vi "Tree.vi"() -> ()   [LabVIEW 2020, in "Nominal Client.lvclass"]
uses:
  Nominal Client.lvclass
  Nominal Client.lvclass/Nominal Client.ctl
  76682c19-609f-4d4f-aff0-eacf46784d00.vi
  2ed37eeb-a64f-4a91-b3eb-4b67bea1485f.vi
  95585ae7-5aba-4d79-b365-cf4aec99f37a.vi
  384434fe-2914-4816-8bdb-9cb29dce40f3.vi
panel:
  in  "Stop wait":bool
  in  "Description":string
  in  "Timestamp Column Name":string
  in  "Dataset Name":string
  in  "File Path":path
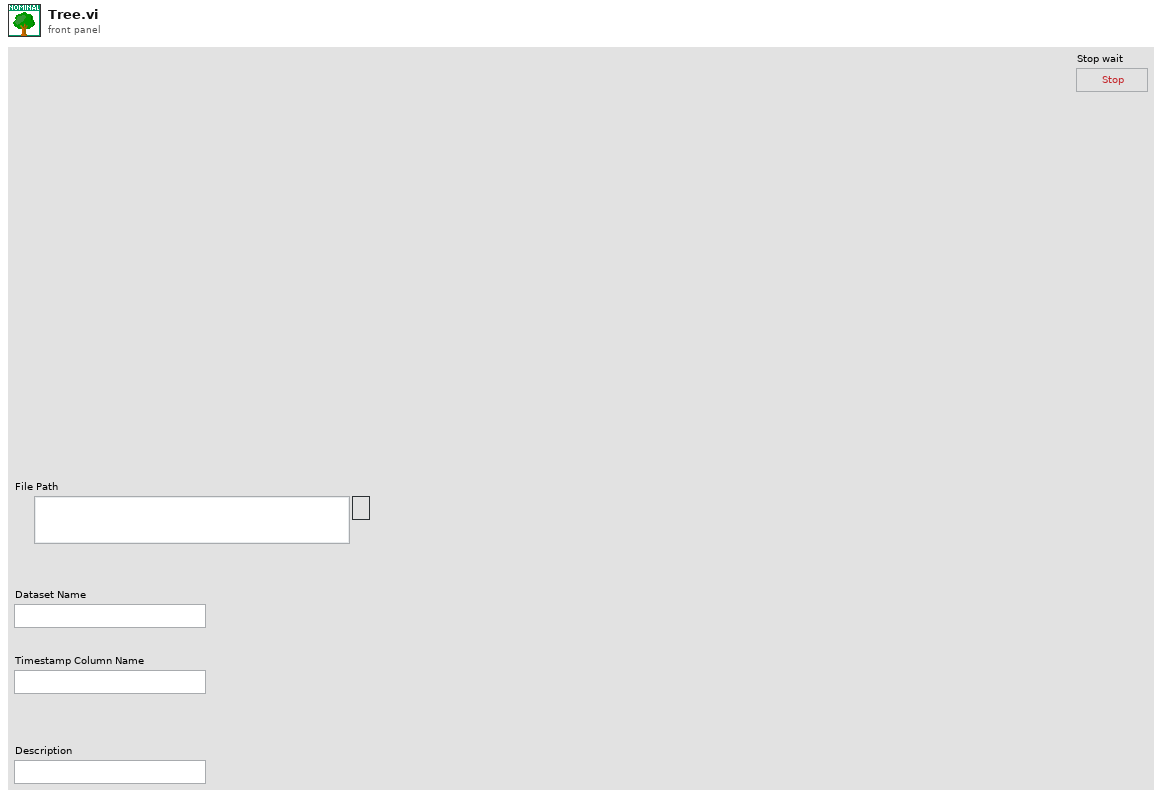
[diagram p1: front panel]
types:
  T1 = cluster{"Channel":string, "Points":cluster{"UNIX Timestamp":cluster{"Seconds":i64, "Nanoseconds":i64}, "Value":string}[]}
  T2 = cluster{"Channel":string, "Points":cluster{"UNIX Timestamp":cluster{"Seconds":i64, "Nanoseconds":i64}, "Value":dbl}[]}
  T3 = enum16{"open", "replace", "create", "open or create", "replace or create", "replace or create with confirmation"}
  T4 = cluster{"datasetRid":string, "datasetFileId":string, "asyncHandle":cluster{"rid":string}}
  T5 = cluster{"Part Number":i32, "ETag":string, "Size":i32}[]
  T6 = cluster{"Channel":string, "Points":cluster{"UNIX Timestamp":cluster{"Seconds":i64, "Nanoseconds":i64}, "Value":dbl}[]}[]
  T7 = cluster{"Channel":string, "Points":cluster{"UNIX Timestamp":cluster{"Seconds":i64, "Nanoseconds":i64}, "Value":string}[]}[]
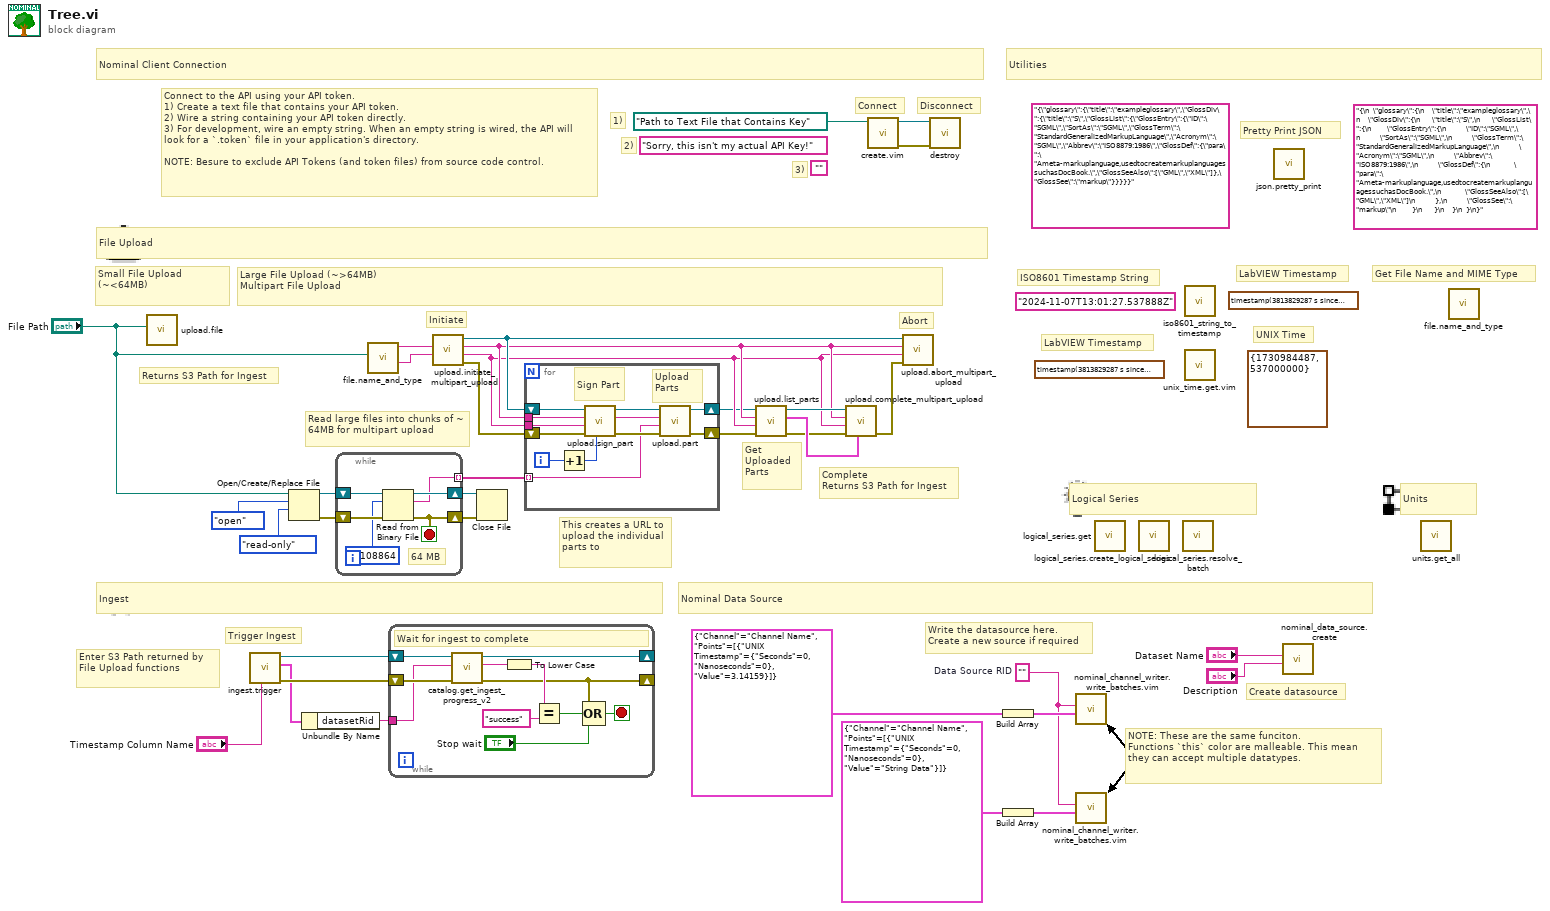
[diagram p0: block diagram]
diagram:
  (unwired) ""
  (unwired) "Sorry, this isn't my actual API Key!" ("API Token (string or path)")
  w9 = ""  # Data Source RID
  (unwired) cluster{"Seconds":i32, "Nanoseconds":i32} {"Seconds"=1730984487, "Nanoseconds"=537000000} ("UNIX Timestamp")
  (unwired) timestamp(3813829287.537 s since 1904-01-01) ("Time Stamp")
  (unwired) timestamp(3813829287.537 s since 1904-01-01) ("Time Stamp")
  (unwired) "2024-11-07T13:01:27.537888Z" ("ISO8601 Timestamp String")
  (unwired) "{\n  \"glossary\":{\n    \"title\":\"exampleglossary\",\n    \"GlossDiv\":{\n      \"title\":\"S\",\n      \"GlossList\":{\n        \"GlossEntry\":{\n          \"ID\":\"SGML\",\n          \"SortAs\":\"SGML\",\n          \"GlossTerm\":\"StandardGeneralizedMarkupLanguage\",\n          \"Acronym\":\"SGML\",\n          \"Abbrev\":\"ISO8879:1986\",\n          \"GlossDef\":{\n            \"para\":\"Ameta-markuplanguage,usedtocreatemarkuplanguagessuchasDocBook.\",\n            \"GlossSeeAlso\":[\"GML\",\"XML\"]\n          },\n          \"GlossSee\":\"markup\"\n        }\n      }\n    }\n  }\n}"
  (unwired) "{\"glossary\":{\"title\":\"exampleglossary\",\"GlossDiv\":{\"title\":\"S\",\"GlossList\":{\"GlossEntry\":{\"ID\":\"SGML\",\"SortAs\":\"SGML\",\"GlossTerm\":\"StandardGeneralizedMarkupLanguage\",\"Acronym\":\"SGML\",\"Abbrev\":\"ISO8879:1986\",\"GlossDef\":{\"para\":\"Ameta-markuplanguage,usedtocreatemarkuplanguagessuchasDocBook.\",\"GlossSeeAlso\":[\"GML\",\"XML\"]},\"GlossSee\":\"markup\"}}}}}"
  # "Get File Name and MIME Type"
  # "Enter S3 Path returned by File Upload functions"
  # "Ingest"
  # "Pretty Print JSON"
  # "Complete\nReturns S3 Path for Ingest"
  # "Returns S3 Path for Ingest"
  # "This creates a URL to upload the individual parts to"
  # "Get Uploaded Parts"
  # "Abort"
  # "Initiate"
  # "Create datasource"
  # "Trigger Ingest"
  # "Disconnect"
  # "Connect"
  # "3)"
  # "2)"
  # "1)"
  # "Connect to the API using your API token.\n1) Create a text file that contains your API token.\n2) Wire a string containing your API token directly.\n3) For development, wire an empty string. When an empty string is wired, the API will look for a `.token` file in your application's directory.\n\nNOTE: Besure to exclude API Tokens (and token files) from source code control."
  # "Nominal Data Source"
  # "NOTE: These are the same funciton.\nFunctions `this` color are malleable. This mean they can accept multiple datatypes."
  # "Write the datasource here.\nCreate a new source if required"
  # "Read large files into chunks of ~ 64MB for multipart upload"
  # "Large File Upload (~>64MB)\nMultipart File Upload"
  # "Small File Upload\n(~<64MB)"
  # "File Upload"
  # "Nominal Client Connection"
  # "Units"
  # "Logical Series"
  # "Utilities"
  # "UNIX Time"
  # "LabVIEW Timestamp"
  # "LabVIEW Timestamp"
  # "ISO8601 Timestamp String"
  n1 = call "upload.file.vi"("File"="File Path") -> ()  [unwired: 7 in, 4 out]
  n2 = call "ingest.trigger.vi"("ISO8601 Timestamp Series Name"="Timestamp Column Name") -> ("error out"=w7:errorcluster, "Information"=w5:T4, "Nominal Client out"=w6:refnum<class "Nominal Client.lvclass">)  [unwired: 7 in, 1 out]
  n3 = Open/Create/Replace File(file path (use dialog)="File Path", operation (0:open)=T3."open", access (0:read/write)=enum16{"read/write", "read-only", "write-only"}."read-only") -> (refnum out=w26:refnum<file>, error out=w23:errorcluster)  [unwired: 3 in, 1 out]
  n4 = Unbundle By Name(w5) -> ("datasetRid"=w4:string)
  n5 = while {
    shift-right: [w40] -> w25
    shift-left: w26 -> [w41]
    shift-right: [w38] -> w24
    shift-left: w23 -> [w39]
    tunnel: [w36] -> w22 mode=indexing
    stop <- w38 stop-if-true
    # "64 MB"
    n6 = Read from Binary File(8:w39, 10:67108864 ("count (1)"), 11:w41) -> (0:w38:errorcluster, 2:w36:string, 3:w40:refnum<file>)  [unwired: 3 in, 1 out]
  }
  n7 = call "file.name_and_type.vi"("File Path"="File Path") -> ("File Type"=w18:string, "File Name"=w19:string)  [unwired: 8 in, 1 out]
  n8 = while {
    shift-right: [w50] -> _
    shift-left: w6 -> [w52]
    shift-right: [w45] -> _
    shift-left: w7 -> [w51]
    tunnel: w4 -> [w49]
    stop <- w42 stop-if-true
    # "Wait for ingest to complete"
    n9 = call "catalog.get_ingest_progress_v2.vi"("error in"=w51, "datasetRid"=w49, "Nominal Client in"=w52) -> ("error out"=w45:errorcluster, "Status"=w48:string, "Nominal Client out"=w50:refnum<class "Nominal Client.lvclass">)  [unwired: 5 in, 1 out]
    n10 = To Lower Case(string=w48) -> (all lower case string=w46:string)
    n11 = Equal?(x=w46, y="success") -> (x = y?=w44:bool)
    n12 = Compound Arithmetic op=OR(w45, w44, "Stop wait") -> (w42:bool)
  }
  n13 = call "upload.initiate_multipart_upload.vi"("File Type"=w18, "File Name"=w19) -> ("error out"=w29:errorcluster, "Key"=w31:string, "Upload ID"=w32:string, "Nominal Client out"=w35:refnum<class "Nominal Client.lvclass">)  [unwired: 6 in]
  n14 = Close File(refnum=w25, error in=w24) -> ()  [unwired: 2 out]
  n15 = for {
    tunnel: w32 -> [w63]
    tunnel: w31 -> [w62]
    shift-right: [w60] -> w30
    shift-left: w35 -> [w64]
    shift-right: [w57] -> w28
    shift-left: w29 -> [w58]
    tunnel: w22 -> [w55] mode=indexing
    i -> [w53]
    # "Sign Part"
    # "Upload\nParts"
    n16 = Increment(x=w53) -> (x+1=w54:i32)
    n17 = call "upload.sign_part.vi"("Part Number"=w54, "error in"=w58, "Key"=w62, "Upload ID"=w63, "Nominal Client in"=w64) -> ("error out"=w56:errorcluster, "url"=w59:string, "Nominal Client out"=w61:refnum<class "Nominal Client.lvclass">)  [unwired: 3 in, 1 out]
    n18 = call "upload.part.vi"("error in"=w56, "Body"=w55, "Path"=w59, "Nominal Client in"=w61) -> ("error out"=w57:errorcluster, "Nominal Client out"=w60:refnum<class "Nominal Client.lvclass">)  [unwired: 5 in, 1 out]
  }
  n19 = call "upload.list_parts.vi"("error in"=w28, "Key"=w31, "Upload ID"=w32, "Nominal Client in"=w30) -> ("error out"=w27:errorcluster, "Parts"=w34:T5, "Nominal Client out"=w33:refnum<class "Nominal Client.lvclass">)  [unwired: 5 in]
  n20 = call "upload.complete_multipart_upload.vi"("Parts"=w34, "error in"=w27, "Key"=w31, "Upload ID"=w32, "Nominal Client in"=w33) -> ("error out"=w16:errorcluster)  [unwired: 4 in, 2 out]
  n21 = call "create.vim"("API Token (string or path)"=path "Path to Text File that Contains Key") -> ("error out"=w14:errorcluster, "Nominal Client"=w15:refnum<class "Nominal Client.lvclass">)  [unwired: 9 in]
  n22 = call "upload.abort_multipart_upload.vi"("error in"=w16, "Key"=w31, "Upload ID"=w32, "Nominal Client in"=w35) -> ()  [unwired: 5 in, 3 out]
  n23 = call "destroy.vi"("error in"=w14, "Nominal Client"=w15) -> ()  [unwired: 9 in, 1 out]
  n24 = Build Array(T2 {"Channel"="Channel Name", "Points"=[{"UNIX Timestamp"={"Seconds"=0, "Nanoseconds"=0}, "Value"=3.14159}]}) -> (w12:T6)
  n25 = Build Array(T1 {"Channel"="Channel Name", "Points"=[{"UNIX Timestamp"={"Seconds"=0, "Nanoseconds"=0}, "Value"="String Data"}]}) -> (w10:T7)
  n26 = call "nominal_channel_writer.write_batches.vim"("batches"=w12, "Data Source RID"=w9) -> ()  [unwired: 6 in, 4 out]
  n27 = call "nominal_channel_writer.write_batches.vim"("batches"=w10, "Data Source RID"=w9) -> ()  [unwired: 6 in, 4 out]
  n28 = call "logical_series.get.vi"() -> ()  [unwired: 8 in, 4 out]
  n29 = call "logical_series.create_logical_series.vi"() -> ()  [unwired: 8 in, 4 out]
  n30 = call "logical_series.resolve_batch.vi"() -> ()  [unwired: 8 in, 4 out]
  n31 = call "iso8601_string_to_timestamp.vi"() -> ()  [unwired: 10 in, 2 out]
  n32 = call "unix_time.get.vim"() -> ()  [unwired: 11 in, 1 out]
  n33 = call "json.pretty_print.vi"() -> ()  [unwired: 10 in, 2 out]
  n34 = call "nominal_data_source.create.vi"("Description"="Description", "ID"="Dataset Name") -> ()  [unwired: 5 in, 5 out]
  n35 = call "units.get_all.vi"() -> ()  [unwired: 8 in, 4 out]
  n36 = call "file.name_and_type.vi"() -> ()  [unwired: 9 in, 3 out]
